vi "Test CVT API.vi"() -> ()   [LabVIEW 2016]
doc: "CVT API Tester."
uses:
  CVT.lvlib
  <vilib>/Utility/error.llb/DialogType.ctl
  <vilib>/Utility/miscctls.llb/LVPointTypeDef.ctl
  Input Command.ctl
panel:
  in  "REQ Initializ CVT":bool
  in  "REQ Write AO Data":bool
  in  "DAQ Type":enum16{"Hardware", "Simulation"}(ring)
  in  "Command":T1
  in  "REQ DC PWS Connect":bool
  in  "Show Diagram on Init":bool
  in  "Show Block Diagram":bool
  in  "Stop Module":bool
  in  "Start Module":bool
  in  "Hide Module Panel":bool
  in  "Show Module Panel":bool
  out "Status":string
  out "Module Running?":bool
  # "This VI tests the API for the Module."
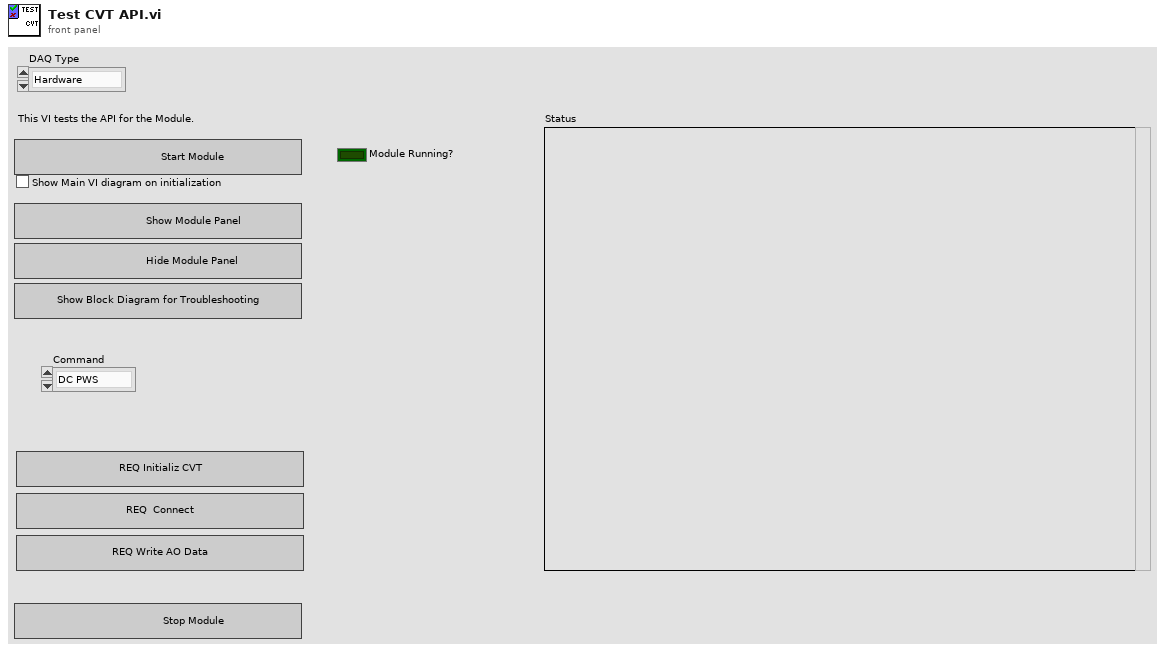
[diagram p1: front panel]
types:
  T1 = typedef "CVT.lvlib/Input Command.ctl" = enum16{"DC PWS", "DMM", "FGEN", "Oscill", "NI DAQ", "NI DIO", "NI CAN", "ESPEC", "ARINC", "MATRIX", "CVT", "Serial"}
  T2 = typedef "LVPointTypeDef.ctl" = cluster{"Horizontal":i16, "Vertical":i16}
  T3 = typedef "CVT.lvlib/Broadcast Events--cluster.ctl" = cluster{"Module Did Init":refnum<user-event>, "Status Updated":refnum<user-event>, "Error Reported":refnum<user-event>, "Module Did Stop":refnum<user-event>, "Update Module Execution Status":refnum<user-event>}
  T4 = typedef "DialogType.ctl" = u16
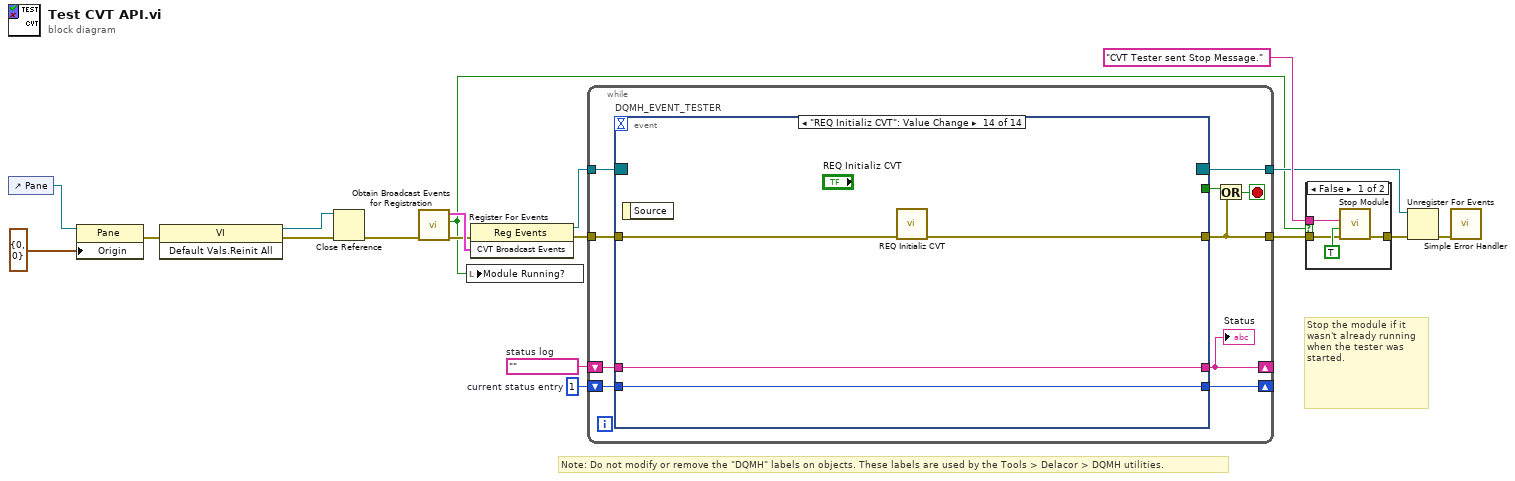
[diagram p0: block diagram]
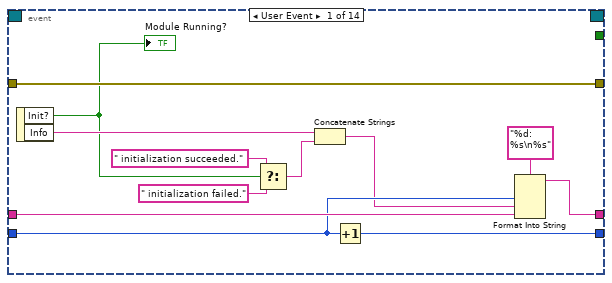
[diagram p3: hidden frame]
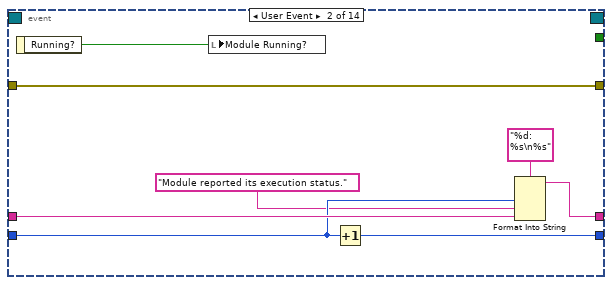
[diagram p4: hidden frame]
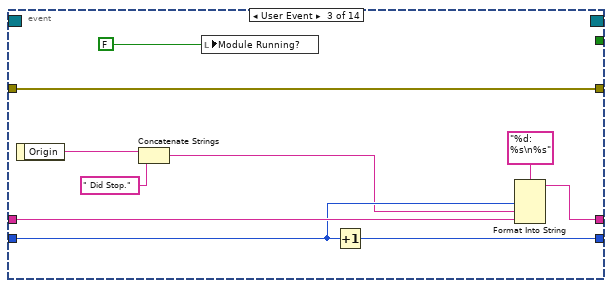
[diagram p5: hidden frame]
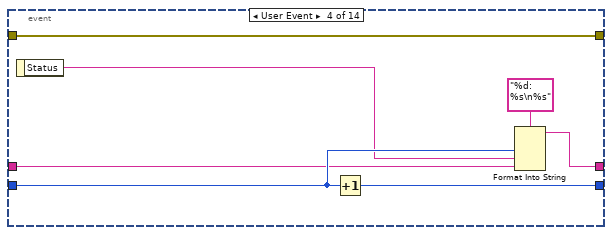
[diagram p6: hidden frame]
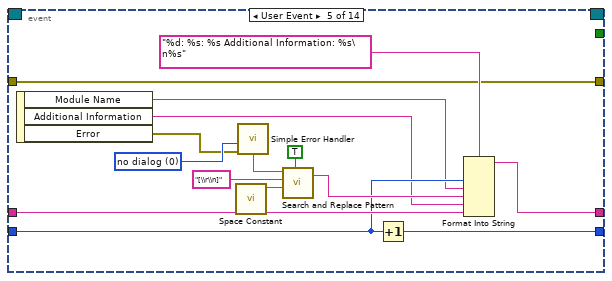
[diagram p7: hidden frame]
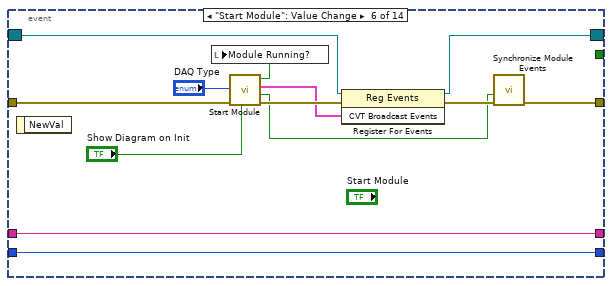
[diagram p8: hidden frame]
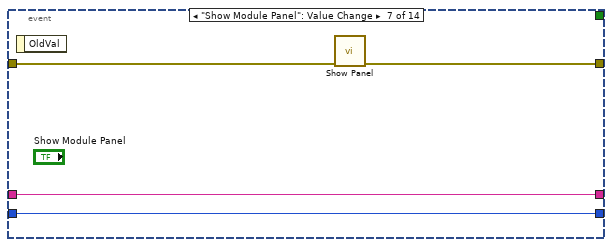
[diagram p9: hidden frame]
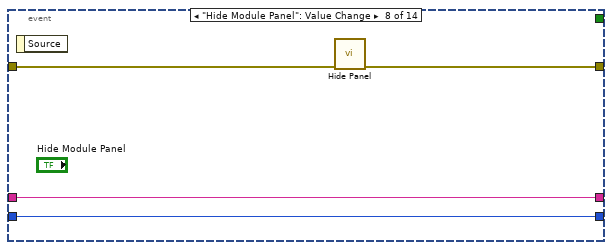
[diagram p10: hidden frame]
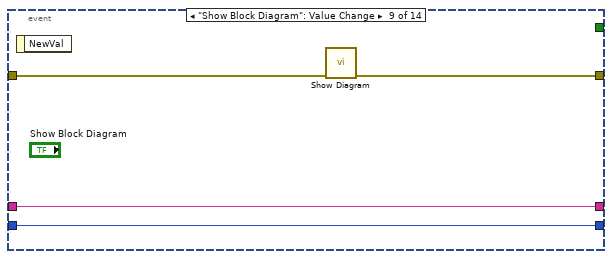
[diagram p11: hidden frame]
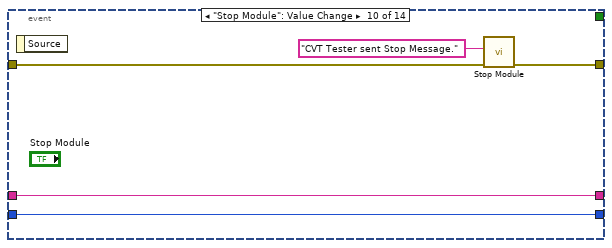
[diagram p12: hidden frame]
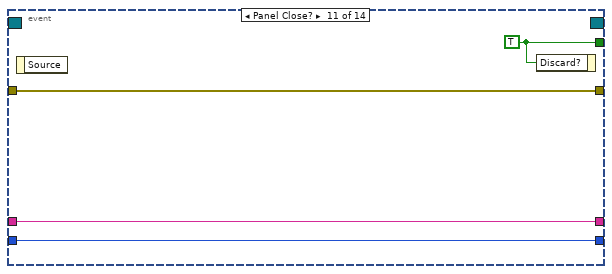
[diagram p13: hidden frame]
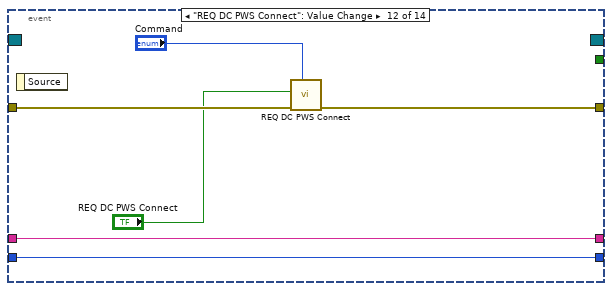
[diagram p14: hidden frame]
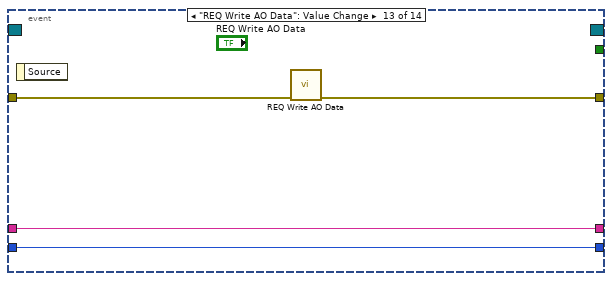
[diagram p15: hidden frame]
diagram:
  w15 = 1  # current status entry
  w16 = ""  # status log
  # "Stop the module if it wasn't already running when the tester was started."
  # "Note: Do not modify or remove the \"DQMH\" labels on objects. These labels are used by the Tools > Delacor > DQMH utilities."
  n1 = control-ref of="Pane"() -> (w3:refnum<vi>)
  n2 = property class="Pane"(reference=w3, "Origin"=T2 {"Horizontal"=0, "Vertical"=0}) -> (error out=w1:errorcluster)  [unwired: 1 in, 1 out]
  n3 = invoke class="VI" method="Default Vals.Reinit All"(error in=w1) -> (reference out=w4:refnum<vi>, error out=w10:errorcluster)  [unwired: 2 in, 1 out]
  n4 = Close Reference(reference=w4, error in (no error)=w10) -> (error out=w5:errorcluster)
  n5 = call "Obtain Broadcast Events for Registration.vi"("error in"=w5) -> ("error out"=w9:errorcluster, "Already running?"=w8:bool, "CVT Broadcast Events"=w13:T3)  [unwired: 8 in]
  n6 = local write "Module Running?"(w8) -> ()
  n7 = register-events(error in=w9, w13) -> (reference out=w12:refnum<event-registration>, error out=w14:errorcluster)  [unwired: 1 in]
  n8 = while {
    tunnel: w12 -> [w28]
    tunnel: [w19] -> w7
    shift-right: [w23] -> _
    shift-left: w16 -> [w25]
    shift-right: [w24] -> _
    shift-left: w15 -> [w26]
    tunnel: w14 -> [w21]
    tunnel: [w20] -> w11
    stop <- w22 stop-if-true
    n9 = event "DQMH_EVENT_TESTER" shown="[13] \"REQ Initializ CVT\": Value Change" {
      selector: w28 -> [_ _ _ _ _ w87 _ _ _ _ _ _ _ _]
      dyn-events: [_ _ _ _ _ w86 _ _ _ _ _ _ _ _] -> w20
      timeout: _ -> [_ _ _ _ _ _ _ _ _ _ _ _ _ _]
      tunnel: [_ _ _ _ _ _ _ _ _ _ w114 _ _ _] -> w27
      tunnel: [w40 w42 w49 w59 w69 w85 w97 w101 w102 w108 w111 w117 w121 w125] -> w19
      tunnel: w26 -> [w37 w46 w56 w62 w72 w90 w95 w99 w103 w109 w112 w118 w122 w126]
      tunnel: w25 -> [w38 w47 w57 w61 w73 w91 w96 w100 w104 w110 w113 w119 w123 w127]
      tunnel: [w35 w44 w54 w63 w71 w91 w96 w100 w104 w110 w113 w119 w123 w127] -> w23
      tunnel: [w36 w45 w55 w65 w70 w90 w95 w99 w103 w109 w112 w118 w122 w126] -> w24
      tunnel: w21 -> [w40 w42 w49 w59 w69 w84 w94 w98 w105 w106 w111 w120 w124 w128]
      event User Event {
        n10 = event-data() -> ("Init?"=w32:bool, "Info"=w34:string)  [unwired: 1 in]
        "Module Running?" <- w32
        n11 = Select(t=" initialization succeeded.", s=w32, f=" initialization failed.") -> (s? t:f=w29:string)
        n12 = Concatenate Strings(w34, w29) -> (w33:string)
        n13 = Increment(x=w37) -> (x+1=w36:i32)
        n14 = Format Into String(format string="%d: %s\n%s", w37, w33, w38) -> (resulting string=w35:string)  [unwired: 2 in, 1 out]
      }
      event User Event {
        n15 = event-data() -> ("Running?"=w41:bool)  [unwired: 1 in]
        n16 = local write "Module Running?"(w41) -> ()
        n17 = Increment(x=w46) -> (x+1=w45:i32)
        n18 = Format Into String(format string="%d: %s\n%s", w46, "Module reported its execution status.", w47) -> (resulting string=w44:string)  [unwired: 2 in, 1 out]
      }
      event User Event {
        n19 = event-data() -> ("Origin"=w53:string)  [unwired: 1 in]
        n20 = Concatenate Strings(w53, " Did Stop.") -> (w52:string)
        n21 = local write "Module Running?"(FALSE ("Module Did Init?")) -> ()
        n22 = Increment(x=w56) -> (x+1=w55:i32)
        n23 = Format Into String(format string="%d: %s\n%s", w56, w52, w57) -> (resulting string=w54:string)  [unwired: 2 in, 1 out]
      }
      event User Event {
        n24 = event-data() -> ("Status"=w60:string)  [unwired: 1 in]
        n25 = Increment(x=w62) -> (x+1=w65:i32)
        n26 = Format Into String(format string="%d: %s\n%s", w62, w60, w61) -> (resulting string=w63:string)  [unwired: 2 in, 1 out]
      }
      event User Event {
        w74 = T4 0 items=["no dialog", "OK message", "continue or stop message", "OK message + warnings", "continue/stop + warnings"] ("type of dialog (OK msg:1)")
        n27 = event-data() -> ("Module Name"=w68:string, "Additional Information"=w67:string, "Error"=w66:errorcluster)  [unwired: 1 in]
        n28 = call <vilib>:"Space Constant.vi"() -> ("String"=w78:string)
        n29 = call <vilib>:"Simple Error Handler.vi"("type of dialog (OK msg:1)"=w74, "error in (no error)"=w66) -> ("message"=w75:string)  [unwired: 3 in, 4 out]
        n30 = call <vilib>:"Search and Replace Pattern.vi"("string"=w75, "regular expression (\"\")"="[\\r\\n]" ("regular expression (\"\")"), "replace string (\"\")"=w78, "replace all? (F)"=TRUE ("replace all CR/LF with spaces")) -> ("result string"=w76:string)  [unwired: 1 in, 1 out]
        n31 = Increment(x=w72) -> (x+1=w70:i32)
        n32 = Format Into String(format string="%d: %s: %s Additional Information: %s\n%s", w72, w68, w76, w67, w73) -> (resulting string=w71:string)  [unwired: 2 in, 1 out]
      }
      event "Start Module": Value Change {
        n33 = event-data() -> ()  [unwired: 1 in, 1 out]
        n34 = call "Start Module.vi"("Show Main VI Diagram on Init (F)"="Show Diagram on Init", "error in"=w84, "DAQ Type"="DAQ Type") -> ("error out"=w92:errorcluster, "Wait for Event Sync?"=w89:bool, "CVT Broadcast Events"=w88:T3, "Module Was Already Running?"=w83:bool)  [unwired: 5 in]
        n35 = local write "Module Running?"(w83) -> ()
        n36 = register-events(reference=w87, error in=w92, w88) -> (reference out=w86:refnum<event-registration>, error out=w93:errorcluster)
        n37 = call "Synchronize Module Events.vi"("error in"=w93, "Wait for Event Sync?"=w89) -> ("error out"=w85:errorcluster)  [unwired: 9 in]
      }
      event "Show Module Panel": Value Change {
        n38 = event-data() -> ()  [unwired: 1 in, 1 out]
        n39 = call "Show Panel.vi"("error in (no error)"=w94) -> ("error out"=w97:errorcluster)  [unwired: 10 in]
      }
      event "Hide Module Panel": Value Change {
        n40 = event-data() -> ()  [unwired: 1 in, 1 out]
        n41 = call "Hide Panel.vi"("error in (no error)"=w98) -> ("error out"=w101:errorcluster)  [unwired: 10 in]
      }
      event "Show Block Diagram": Value Change {
        n42 = event-data() -> ()  [unwired: 1 in, 1 out]
        n43 = call "Show Diagram.vi"("error in (no error)"=w105) -> ("error out"=w102:errorcluster)  [unwired: 10 in]
      }
      event "Stop Module": Value Change {
        n44 = event-data() -> ()  [unwired: 1 in, 1 out]
        n45 = call "Stop Module.vi"("error in"=w106, "Origin"="CVT Tester sent Stop Message.") -> ("error out"=w108:errorcluster)  [unwired: 9 in]
      }
      event Panel Close? {
        w114 = TRUE ("Discard?")
        n46 = event-data() -> ()  [unwired: 1 in, 1 out]
        n47 = event-data("Discard?"=w114) -> ()  [unwired: 1 in, 1 out]
      }
      event "REQ DC PWS Connect": Value Change {
        n48 = event-data() -> ()  [unwired: 1 in, 1 out]
        n49 = call "REQ DC PWS Connect.vi"("Command"="Command", "error in"=w120, "Connect ?"="REQ DC PWS Connect") -> ("error out"=w117:errorcluster)  [unwired: 8 in]
      }
      event "REQ Write AO Data": Value Change {
        n50 = event-data() -> ()  [unwired: 1 in, 1 out]
        n51 = call "REQ Write AO Data.vi"("error in"=w124) -> ("error out"=w121:errorcluster)  [unwired: 10 in]
      }
      event "REQ Initializ CVT": Value Change {
        n52 = event-data() -> ()  [unwired: 1 in, 1 out]
        n53 = call "REQ Initializ CVT.vi"("error in"=w128) -> ("error out"=w125:errorcluster)  [unwired: 8 in, 2 out]
      }
    }
    "Status" <- w23
    n54 = Or(x=w27, y=w19) -> (x .or. y?=w22:bool)
  }
  n55 = case shown="False" w8 {
    tunnel: [w132 w133] -> w18
    tunnel: "CVT Tester sent Stop Message." ("Origin") -> [w131 _]
    tunnel: w7 -> [w129 w133]
    frame False {
      n56 = call "Stop Module.vi"("error in"=w129, "Wait for Module to Stop? (F)"=TRUE ("Wait for Module to stop?"), "Origin"=w131) -> ("error out"=w132:errorcluster)  [unwired: 8 in]
    }
    frame True {
    }
  }
  n57 = Unregister For Events(event registration refnum=w11, error in=w18) -> (error out=w6:errorcluster)
  n58 = call <vilib>:"Simple Error Handler.vi"("error in (no error)"=w6) -> ()  [unwired: 4 in, 5 out]
